vi "libssh2_session_last_error.vi"(8 "error in (no error)":errorcluster, 11 "session":u64) -> (0 "error out":errorcluster, 2 "errmsg":string, 3 "return value":i32)   [LabVIEW 2013, in "libssh2.lvlib"]
uses:
  libssh2.lvlib
  libssh2.dll
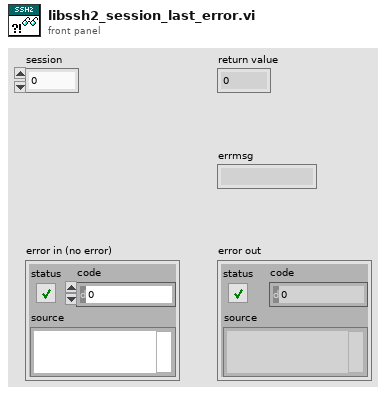
[diagram p1: front panel]
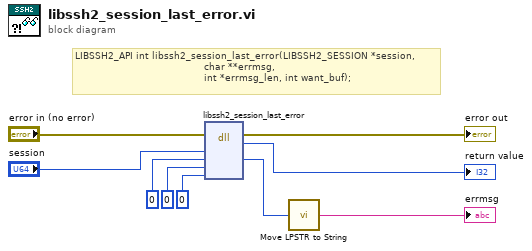
[diagram p0: block diagram]
diagram:
  # "LIBSSH2_API int libssh2_session_last_error(LIBSSH2_SESSION *session,\n                                           char **errmsg,\n                                           int *errmsg_len, int want_buf);"
  n1 = dll-call lib="C:/Users/pasca/source/repos/libssh2-labview/libssh2**.*" fn="libssh2_session_last_error"(error in="error in (no error)", "session"="session", "errmsg"=u64 0, "errmsg_len"=0, "want_buf"=0) -> (error out=→"error out":errorcluster, "return value"=→"return value":i32, "errmsg"=w5:u64)  [unwired: 5 in, 1 out]
  n2 = call "Move LPSTR to String.vi"("LPSTR"=w5) -> ("String"=→"errmsg":string)  [unwired: 1 in]
